vi "Timer Destroy.vi"(8 "error in (no error)":errorcluster, 11 "Timer reference":refnum<data-value>) -> (0 "error out":errorcluster)   [LabVIEW 2009]
doc: "This VI is part of a Timer class that is implemented with the DVR. It destroys the Timer.\n\nAAL 9/09"
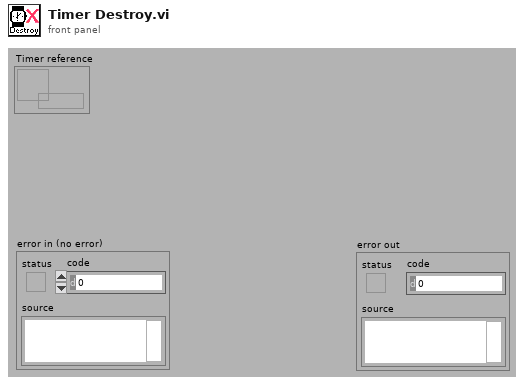
[diagram p1: front panel]
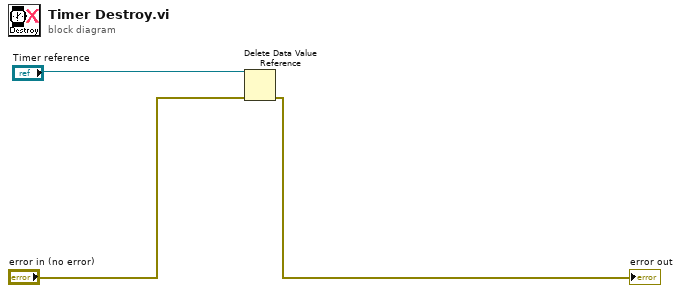
[diagram p0: block diagram]
diagram:
  n1 = Delete Data Value Reference(data value reference="Timer reference", error in="error in (no error)") -> (error out=→"error out":errorcluster)  [unwired: 1 out]
